vi "Example TCP AI.vi"() -> ()   [LabVIEW 2010]
doc: "Illustrates the simplest form of TCP data acquisition using a TCP data server.\n\n\nCreated by Monroe Weber-Shirk\nCornell University\nmw24@cornell.edu\nJanuary 2000"
panel:
  in  "Data Servers":string[](array[string])=["calcium.cee.cornell.edu", "Dataserver.cee.cornell.edu"]
  in  "Scans per Sample":i32=1 min=1
  in  "channel indices":i32[](array[numeric])
  in  "stop":bool
  out "Waveform Chart":sgl[][](graph)
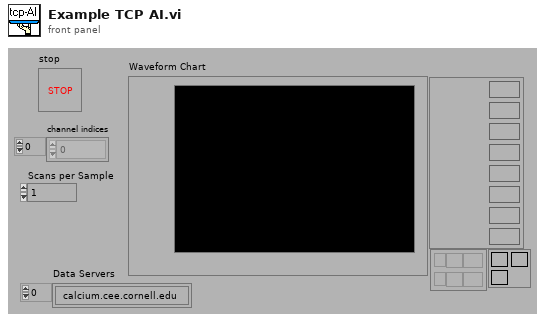
[diagram p1: front panel]
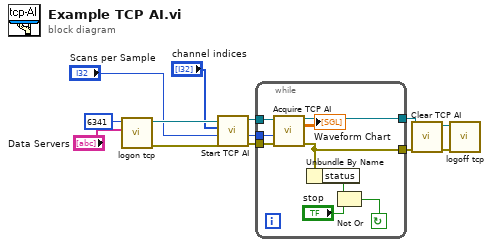
[diagram p0: block diagram]
diagram:
  n1 = call "logon tcp.vi"("Data Servers"="Data Servers", "port"=u16 6341) -> ("error out"=w5:errorcluster, "connection ID"=w13:refnum<k5>)  [unwired: 4 in, 4 out]
  n2 = call "Start TCP AI.vi"("error in (no error)"=w5, "Scans per Sample"="Scans per Sample", "channel indices"="channel indices", "Connection ID in"=w13) -> ("error out"=w3:errorcluster, "channels"=w8:i32, "Connection ID out"=w12:refnum<k5>)  [unwired: 5 in]
  n3 = while {
    tunnel: [w14] -> w2
    tunnel: w3 -> [w15]
    tunnel: w8 -> [w16]
    tunnel: [w20] -> w11
    tunnel: w12 -> [w21]
    stop <- w17 continue-if-true
    n4 = call "Acquire TCP AI.vi"("connection ID"=w21, "channels"=w16, "error in"=w15) -> ("connection ID out"=w20:refnum<k5>, "voltage data"=→"Waveform Chart":sgl[][], "error out"=w14:errorcluster)  [unwired: 8 in, 2 out]
    n5 = Unbundle By Name(w14) -> ("status"=w19:bool)
    n6 = Not Or(1:"stop", 2:w19) -> (0:w17:bool)
  }
  n7 = call "Clear TCP AI.vi"("error in (no error)"=w2, "Connection ID in"=w11) -> ("error out"=w9:errorcluster, "Connection ID out"=w10:refnum<k5>)  [unwired: 8 in]
  n8 = call "logoff tcp.vi"("error in (no error)"=w9, "Connection ID"=w10) -> ()  [unwired: 8 in, 2 out]
